vi "DIAdem Start.vi"(8 "error in":errorcluster, 9 "Init VBS Full Path (empty)":path, 10 "Version String (\"\")":string, 11 "DataFinder (\"\")":string) -> (0 "error out":errorcluster, 2 "DIAdem Desktop File":path, 3 "DIAdem Reference":T1)   [LabVIEW 2011]
uses:
  <vilib>/ExportToExcel/DIAdem Reference.ctl
  Addons/DIAdem/DIAdem.llb/DIAdem String Variable Set.vi
  Addons/DIAdem/DIAdem.llb/DIAdem String Variable Get.vi
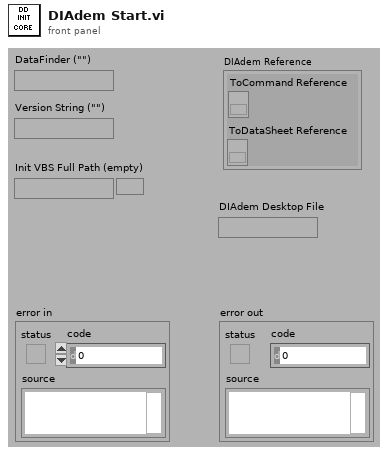
[diagram p1: front panel]
types:
  T1 = typedef "DIAdem Reference.ctl" = cluster{"ToCommand Reference":refnum<k7>, "ToDataSheet Reference":refnum<k7>}
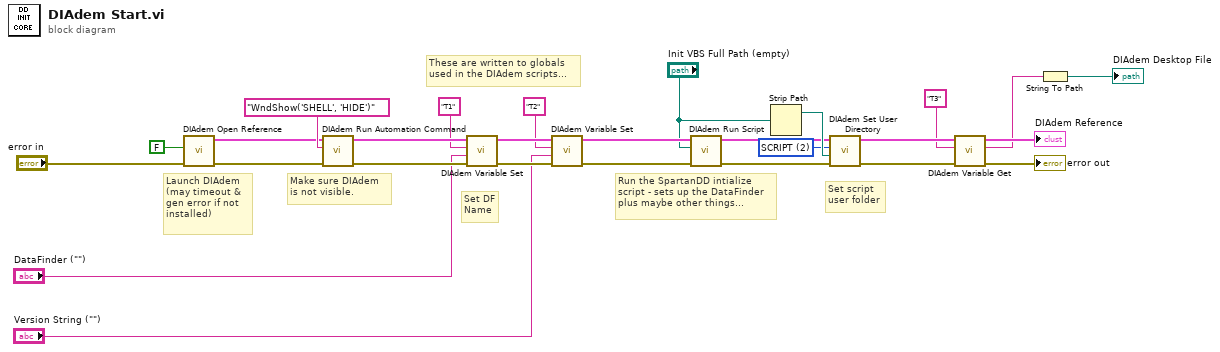
[diagram p0: block diagram]
diagram:
  w23 = u16 2 items=["NAVIGATOR", "REPORT", "SCRIPT"] ("DIAdem panel")
  # "These are written to globals\nused in the DIAdem scripts..."
  # "Set DF\nName"
  # "Run the SpartanDD intialize\nscript - sets up the DataFinder\nplus maybe other things..."
  # "Make sure DIAdem\nis not visible."
  # "Launch DIAdem\n(may timeout &\ngen error if not\ninstalled)"
  # "Set script\nuser folder"
  n1 = call "DIAdem Open Reference.vi"("error in (no error)"="error in", "Show Environment (F)"=FALSE) -> ("error out"=w19:errorcluster, "DIAdem Reference"=w20:T1)  [unwired: 2 in, 6 out]
  n2 = call "DIAdem Run Automation Command.vi"("error in (no error)"=w19, "command"="WndShow('SHELL', 'HIDE')", "DIAdem Reference"=w20) -> ("error out"=w26:errorcluster, "DIAdem Reference"=w25:T1)  [unwired: 7 out]
  n3 = call-poly "DIAdem Variable Set.vi"("error in (no error)"=w26, "Value"="DataFinder (\"\")", "Variable Name"="T1", "DIAdem Reference"=w25) -> ("error out"=w15:errorcluster, "DIAdem Reference"=w13:T1)  [unwired: 6 out]
  n4 = call-poly "DIAdem Variable Set.vi"("error in (no error)"=w15, "Value"="Version String (\"\")", "Variable Name"="T2", "DIAdem Reference"=w13) -> ("error out"=w14:errorcluster, "DIAdem Reference"=w12:T1)  [unwired: 6 out]
  n5 = call "DIAdem Run Script.vi"("error in (no error)"=w14, "script file"="Init VBS Full Path (empty)", "DIAdem Reference"=w12) -> ("error out"=w17:errorcluster, "DIAdem Reference"=w18:T1)  [unwired: 7 out]
  n6 = Strip Path(path="Init VBS Full Path (empty)") -> (stripped path=w27:path)  [unwired: 1 out]
  n7 = call "DIAdem Set User Directory.vi"("error in (no error)"=w17, "user directory"=w27, "DIAdem panel"=w23, "DIAdem Reference"=w18) -> ("error out"=w7:errorcluster, "DIAdem Reference"=w5:T1)  [unwired: 6 out]
  n8 = call-poly "DIAdem Variable Get.vi"("error in (no error)"=w7, "Variable Name"="T3", "DIAdem Reference"=w5) -> ("error out"=→"error out":errorcluster, "Value"=w2:string, "DIAdem Reference"=→"DIAdem Reference":T1)  [unwired: 6 out]
  n9 = String To Path(string=w2) -> (path=→"DIAdem Desktop File":path)
